vi "signal_values_FGV.vi"(0 "Action":T3, 1 "Hz Value":dbl, 2 "Waveform":T2(ring), 3 "Offset":dbl, 5 "Amp String":string, 7 "Hz String":string, 9 "Amp Value":dbl, 11 "Error In":errorcluster, 12 "Phase":dbl) -> (4 "Signal":T1, 15 "Error Out":errorcluster)   [LabVIEW 2021, in "Signal.lvlib"]
doc: "This FGV is used to memorize and operate with the signal properties."
uses:
  Signal.lvlib
  Tipski Definicii/Signal Values.ctl
  <vilib>/measure/NI_MABase.lvlib
panel:
  # "Output"
  # "Input"
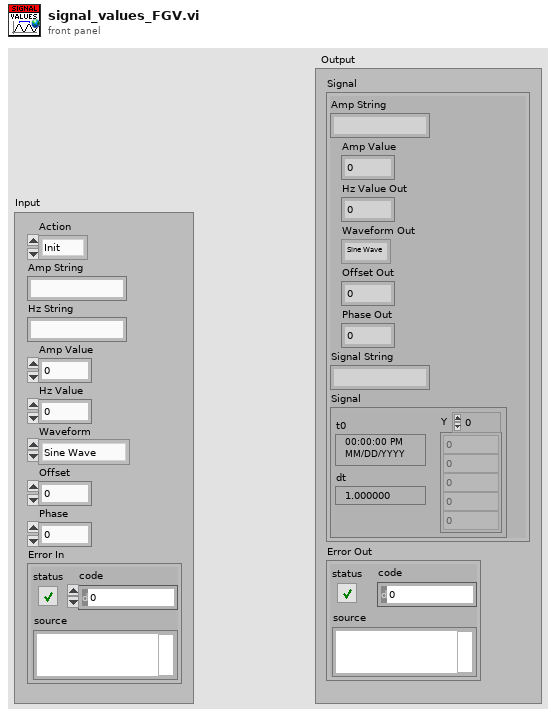
[diagram p1: front panel]
types:
  T1 = cluster{"Amp String":string, "Amp Value":dbl, "Hz Value Out":dbl, "Waveform Out":enum16{"Sine Wave", "Triangle Wave", "Square Wave", "Sawtooth Wave"}, "Offset Out":dbl, "Phase Out":dbl, "Signal String":string, "Signal":waveform(dbl)}
  T2 = enum16{"Sine Wave", "Triangle Wave", "Square Wave", "Sawtooth Wave"}
  T3 = typedef "Signal Values.ctl" = enum16{"Init", "Add V/A string", "Add Hz string", "Get Strings and Values", "Reset", "Add Offset", "Add Waveform", "Add Phase"}
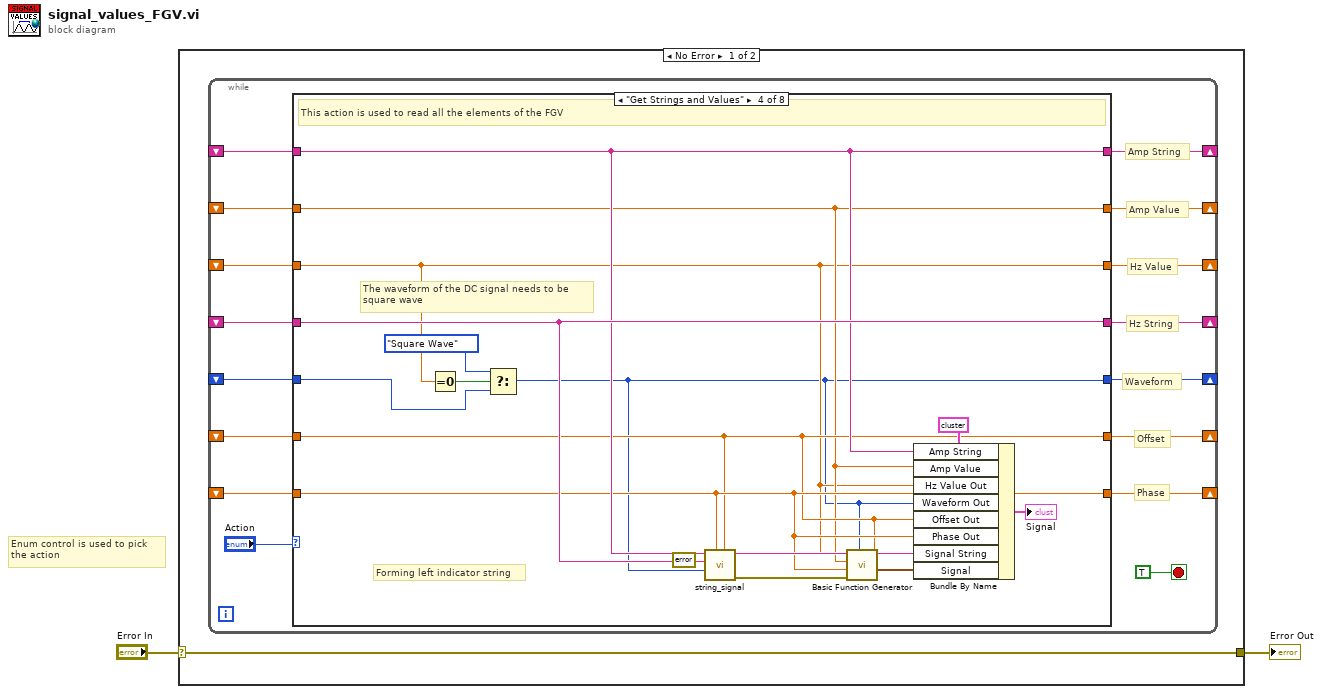
[diagram p0: block diagram]
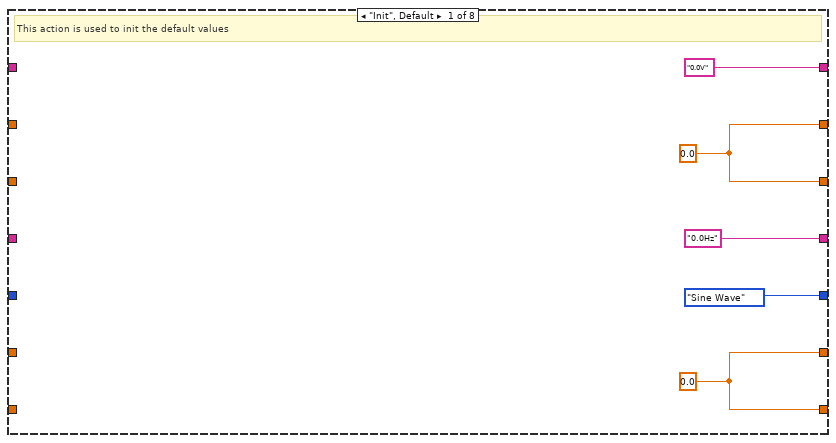
[diagram p2: hidden frame]
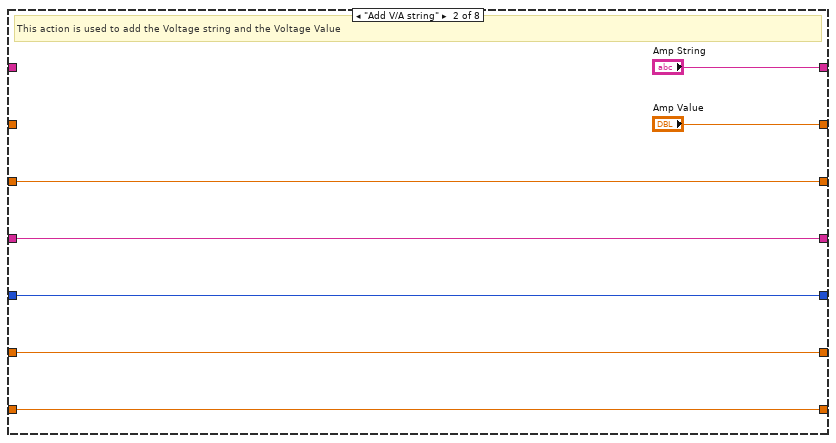
[diagram p3: hidden frame]
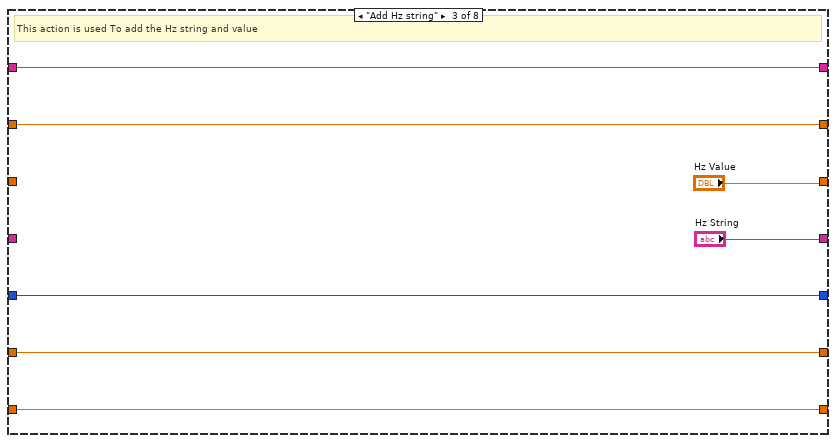
[diagram p4: hidden frame]
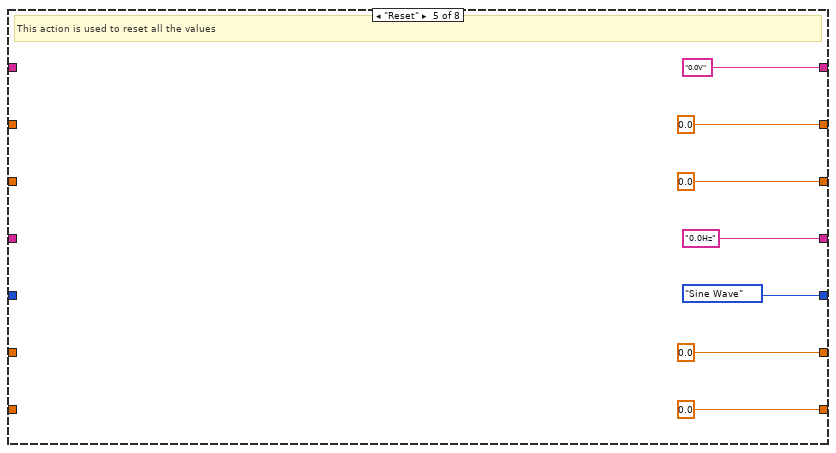
[diagram p5: hidden frame]
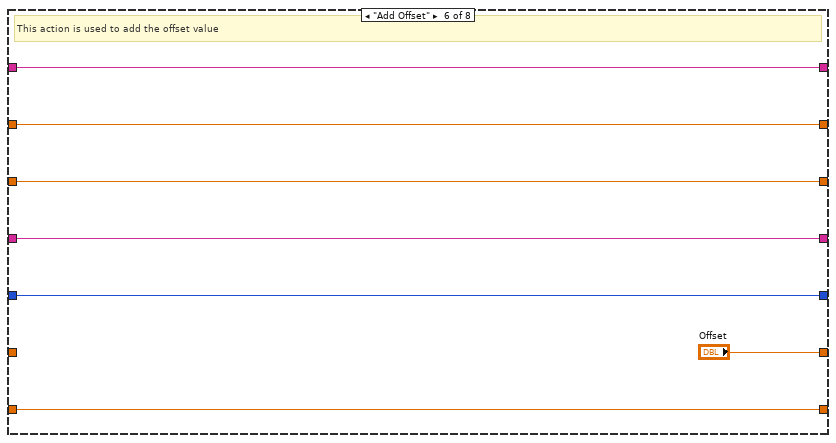
[diagram p6: hidden frame]
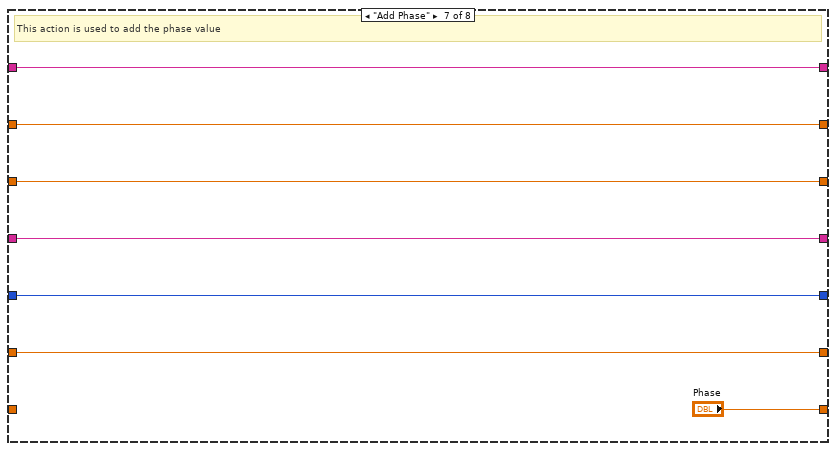
[diagram p7: hidden frame]
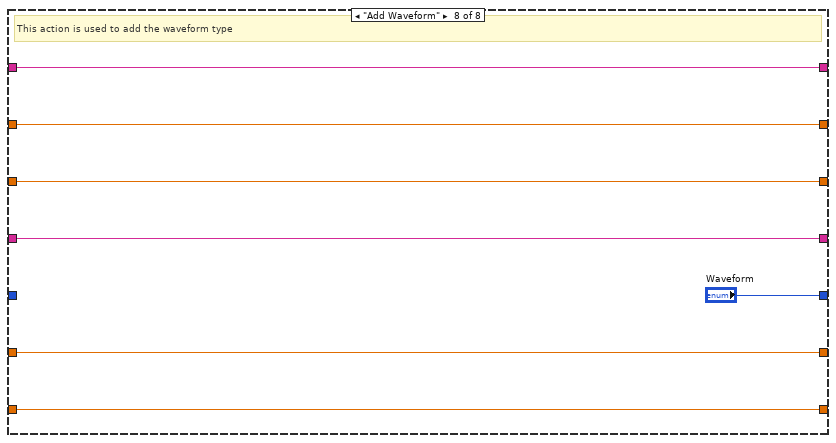
[diagram p8: hidden frame]
diagram:
  # "Enum control is used to pick \nthe action"
  n1 = case shown="No Error" "Error In" {
    selector: "Error In" -> [w3 w83]
    tunnel: [w3 w83] -> w1
    frame No Error {
      n2 = while {
        shift-right: [w17] -> _
        shift-left: _ -> [w13]
        shift-right: [w15] -> _
        shift-left: _ -> [w12]
        shift-right: [w14] -> _
        shift-left: _ -> [w11]
        shift-right: [w16] -> _
        shift-left: _ -> [w10]
        shift-right: [w9] -> _
        shift-left: _ -> [w8]
        shift-right: [w7] -> _
        shift-left: _ -> [w5]
        shift-right: [w6] -> _
        shift-left: _ -> [w4]
        stop <- TRUE stop-if-true
        # "Phase"
        # "Offset"
        # "Waveform"
        # "Hz String"
        # "Hz Value"
        # "Amp Value"
        # "Amp String"
        n3 = case shown="\"Get Strings and Values\"" "Action" {
          tunnel: ["0.0V" "Amp String" w36 w53 "0.0V" ("Voltage String") w68 w75 w78] -> w17
          tunnel: ["0.0Hz" w28 "Hz String" w54 "0.0Hz" ("String") w65 w72 w81] -> w16
          tunnel: [w22 "Amp Value" w35 w44 0.0 ("Voltage Value") w67 w74 w79] -> w15
          tunnel: [w22 w29 "Hz Value" w43 0.0 ("Hz Value") w66 w73 w80] -> w14
          tunnel: w13 -> [_ _ w36 w53 _ w68 w75 w78]
          tunnel: w12 -> [_ _ w35 w44 _ w67 w74 w79]
          tunnel: w11 -> [_ w29 _ w43 _ w66 w73 w80]
          tunnel: w10 -> [_ w28 _ w54 _ w65 w72 w81]
          tunnel: [T2."Sine Wave" ("signal type") w27 w34 w39 T2."Sine Wave" ("signal type") w64 w71 "Waveform"] -> w9
          tunnel: w8 -> [_ w27 w34 w40 _ w64 w71 _]
          tunnel: [w20 w26 w33 w47 0.0 "Offset" w70 w77] -> w7
          tunnel: [w20 w25 w32 w48 0.0 w62 "Phase" w76] -> w6
          tunnel: w5 -> [_ w26 w33 w47 _ _ w70 w77]
          tunnel: w4 -> [_ w25 w32 w48 _ w62 _ w76]
          frame "Init", Default {
            w20 = 0.0
            w22 = 0.0
            # "This action is used to init the default values"
          }
          frame "Add V/A string" {
            # "This action is used to add the Voltage string and the Voltage Value"
          }
          frame "Add Hz string" {
            # "This action is used To add the Hz string and value"
          }
          frame "Get Strings and Values" {
            # "The waveform of the DC signal needs to be \nsquare wave"
            # "Forming left indicator string"
            # "This action is used to read all the elements of the FGV"
            n4 = Equal To 0?(x=w43) -> (x = 0?=w42:bool)
            n5 = Select(t=T2."Square Wave" ("Waveform"), s=w42, f=w40) -> (s? t:f=w39:T2)
            n6 = call "string_signal.vi"("Offset"=w47, "Phase"=w48, "Error In"=errorcluster {"status"=FALSE, "code"=0, "source"=""}, "Waveform"=w39, "Hz String"=w54, "Amp String"=w53) -> ("Error Out"=w49:errorcluster, "Signal String"=w52:string)  [unwired: 4 in]
            n7 = call <vilib>:"Basic Function Generator.vi"("offset"=w47, "signal type"=w39, "error in (no error)"=w49, "phase"=w48, "amplitude"=w44, "frequency"=w43) -> ("signal out"=w45:waveform(dbl))  [unwired: 3 in, 2 out]
            n8 = Bundle By Name(cluster=T1 {"Amp String"="", "Amp Value"=0.0, "Hz Value Out"=0.0, "Waveform Out"=enum."Sine Wave", "Offset Out"=0.0, "Phase Out"=0.0, "Signal String"="", "Signal"={"t0"=timestamp(0 s since 1904-01-01), "dt"=1.0, "Y"=[]}} ("Signal Value Cluster"), "Amp String"=w53, "Amp Value"=w44, "Hz Value Out"=w43, "Waveform Out"=w39, "Offset Out"=w47, "Phase Out"=w48, "Signal String"=w52, "Signal"=w45) -> (→"Signal":T1)
          }
          frame "Reset" {
            # "This action is used to reset all the values"
          }
          frame "Add Offset" {
            # "This action is used to add the offset value"
          }
          frame "Add Phase" {
            # "This action is used to add the phase value"
          }
          frame "Add Waveform" {
            # "This action is used to add the waveform type"
          }
        }
      }
    }
    frame Error {
    }
  }
  "Error Out" <- w1
